vi "Lab5_template_v4.0.vi"() -> ()   [LabVIEW 2018]
doc: "Main VI for the controls"
uses:
  components/PMCL Dynamic Signal Analyzer/Controls/DSA excitation specs.ctl
  components/PMCL Dynamic Signal Analyzer/Controls/DSA cycle specs.ctl
  Typedefs/StateDef_Enum.ctl
  <vilib>/Utility/error.llb/DialogType.ctl
  <vilib>/Platform/TimedLoop/XDataNode/timing_clust.ctl
  <vilib>/Platform/TimedLoop/XDataNode/nitl_modes.ctl
  <vilib>/Platform/TimedLoop/XDataNode/wakeup.ctl
  <vilib>/DAQmx/read.llb/DAQmx Read (Analog 1D DBL NChan 1Samp).vi
  <vilib>/DAQmx/write.llb/DAQmx Write (Analog DBL 1Chan 1Samp).vi
  <vilib>/DAQmx/create/channels.llb/DAQmx Create Channel (AO-Voltage-Basic).vi
  <vilib>/DAQmx/create/channels.llb/DAQmx Create Channel (AI-Voltage-Basic).vi
  <vilib>/DAQmx/configure/timing.llb/DAQmx Timing (Sample Clock).vi
  <vilib>/DAQmx/create/timing.llb/DAQmx Create Timing Source (Control Loop From Task).vi
  <vilib>/DAQmx/miscellaneous.llb/DAQmx Fill In Error Info.vi
  <vilib>/platform/TimedLoop/XDataNode/XDataNode.xnode
  Components/Timing/Timing.lvlib
  <vilib>/Platform/TimedLoop/XDataNode/XDNodeRunTimeDep.lvlib
  <vilib>/Analysis/NI_AALPro.lvlib
  <vilib>/ptbypt/NI_PtbyPt.lvlib
  Components/Controller/Controller.lvlib
panel:
  in  "System Stop Button":bool
  in  "Pause chart?":bool
  in  "Controller Params":enum32{"Page 1"}(tab)
  in  "Kp":dbl=1.0 min=0.0
  in  "Controller On?":bool
  out "Status":string
  in  "Ref. Gen.":enum32{"Analog In", "Manual", "Wave Gen", "DSA"}(tab)=enum."Manual"
  in  "Ref. cmd.":dbl(slide) step=1.0 scale=-10.0..10.0 scale format="%#.1f"
  in  "Signal Cluster":T1={"phase"=0.0, "amplitude"=1.0, "frequency"=1.0, "offset"=1.0, "Signal"=enum."Square"} {"offset" format="%0.2f"; "frequency" format="%0.2f"; "amplitude" format="%0.2f"; "phase" format="%0.2f"}
  in  "Frequency\nResponse":enum16{"Plant", "RR", "CL"}(ring)
  out "DSA \nRunning?":bool
  in  "Stop \nDSA":bool
  in  "Start \nDSA":bool
  in  "DSA excitation specs":T2={"Initial Freq. [Hz]"=10.0, "Final Freq. [Hz]"=999.0, "# pts. in interval"=50, "Samping Time [s]"=0.001, "Amplitude [V]"=1.0, "Offset [V]"=0.0, "Freq Units (F: rad/s, T: Hz)"=TRUE}
  in  "Cycle Specs":T3={"Cycles To \nSettle (M)"=5, "Cycles To \nCalculate (N)"=10}
  in  "Loop Timing":enum32{"Ctrl.", "Ref. gen", "UI"}(tab)
  in  "Ctrl.\nLoop Rate (Hz)":dbl=20000.0 format="%#_4p"
  out "# Finished\nLate counter":dbl
  out "# Finished\nLate counter":dbl
  in  "Ref. Gen.\nLoop Rate (Hz)":dbl=20000.0 format="%#_4p"
  in  "UI Loop rate (Hz)":dbl=1000.0 format="%#_6p"
  in  "Display Waveforms":enum32{"Controller Signals", "DSA "}(tab)
  out "Control Effort":dbl(graph)
  out "Waveform Chart":cluster{"Double":dbl, "Numeric":dbl}(graph)
  out "Phase Bode Plot":cluster{dbl[], dbl[]}(graph)
  out "Magnitude Bode Plot":cluster{dbl[], dbl[]}(graph)
  out "DSA Signals":cluster{"Double":dbl, "Double":dbl}(graph)
  # "Connect the Reference Signal \nto C/AI 1 of the myRIO."
  # "Pinout Config.:\nPort C/AI0 : Plant output being read           by the controller.\nPort C/AI1 : Reference signal for the control loop.\nPort C/AO0 : Control effort signal to the plant."
  # "Control Loop Timing"
  # "Ref.  Gen. Loop Timing"
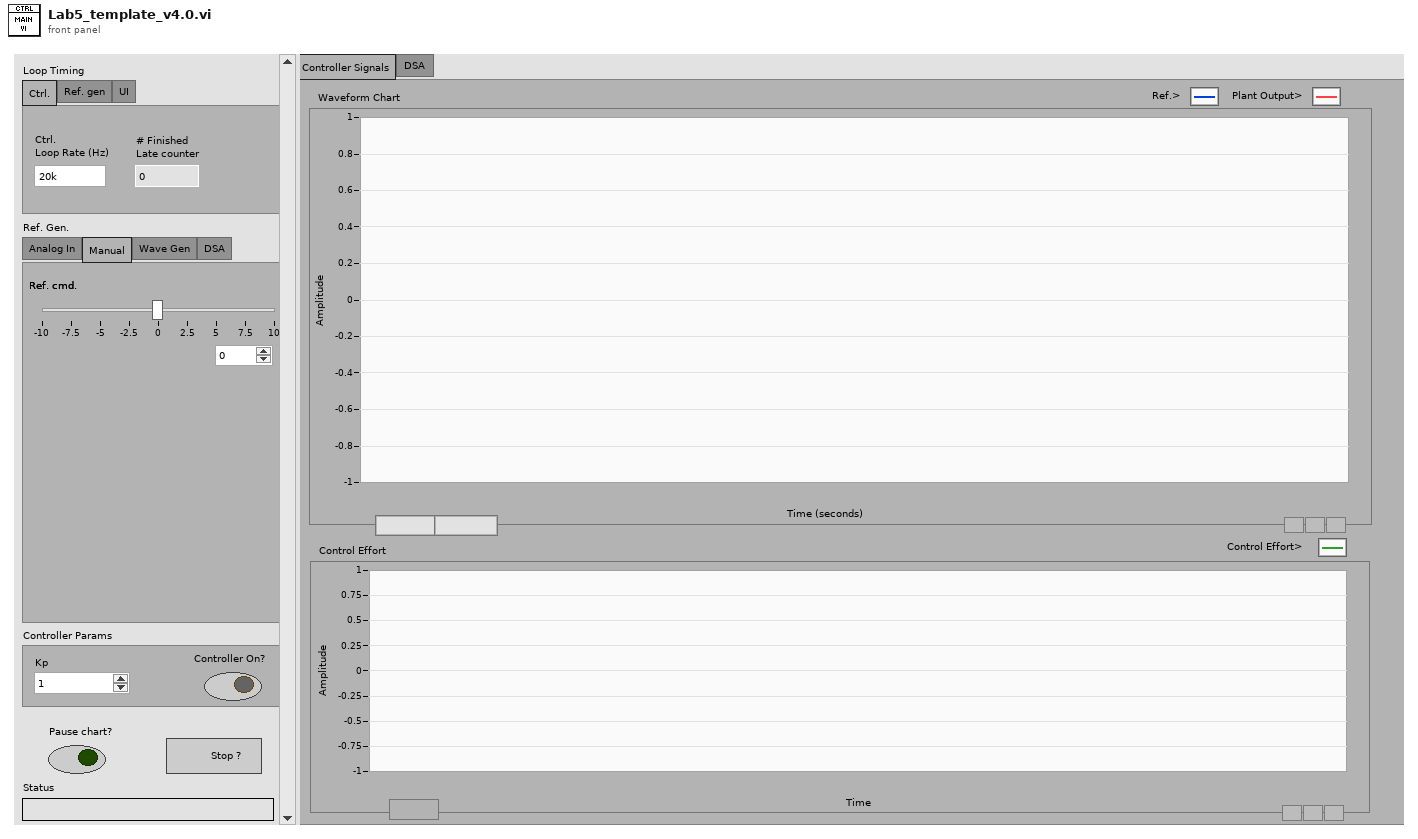
[diagram p1: front panel]
types:
  T1 = cluster{"phase":dbl, "amplitude":dbl, "frequency":dbl, "offset":dbl, "Signal":enum16{"Sine", "Square", "Sawtooth"}}
  T2 = typedef "DSA excitation specs.ctl" = cluster{"Initial Freq. [Hz]":dbl, "Final Freq. [Hz]":dbl, "# pts. in interval":i16, "Samping Time [s]":dbl, "Amplitude [V]":dbl, "Offset [V]":dbl, "Freq Units (F: rad/s, T: Hz)":bool}
  T3 = typedef "DSA cycle specs.ctl" = cluster{"Cycles To \nSettle (M)":i16, "Cycles To \nCalculate (N)":i16}
  T4 = typedef "DialogType.ctl" = u16
  T5 = typedef "StateDef_Enum.ctl" = enum16{"Initialize", "Wait", "Shutdown"}
  T6 = typedef "XDNodeRunTimeDep.lvlib/timing_clust.ctl" = cluster{"Expected End [f-1]":u64, "Actual End [f-1]":u64, "Finished Late? [f-1]":bool, "Expected End [i-1]":u64, "Actual End [i-1]":u64, "Finished Late? [i-1]":bool, "Expected Start [i]":u64, "Actual Start [i]":u64, "Expected Start [f]":u64, "Actual Start [f]":u64, "Source Name":string, "Structure Name":string, "Period":i64, "Deadline":i64, "Offset":i64, "Start":i64, "Priority":i32, "Timeout":i32, "Mode":T7, "Wakeup Reason":T8, "Error":errorcluster, "Source Type":string, "Secondary Source Type":string, "Global End Time":u64, "Global Start Time":u64, "Frame Duration":u64, "Iteration Duration":u64, "Assigned CPU":i32, "I/O Scan Engine Mode":u32}
  T7 = typedef "XDNodeRunTimeDep.lvlib/nitl_modes.ctl" = enum32{"No Change", "Process missed periods, maintain original phase", "Discard missed periods, maintain original phase", "Process missed periods, ignore original phase", "Discard missed periods, ignore original phase"}
  T8 = typedef "XDNodeRunTimeDep.lvlib/wakeup.ctl" = enum32{"Normal", "Aborted", "Asynchronous wakeup", "Timing source error", "Timed loop error", "Timeout"}
  T9 = cluster{"Analog In CH1":dbl, "Analog In CH0":dbl}
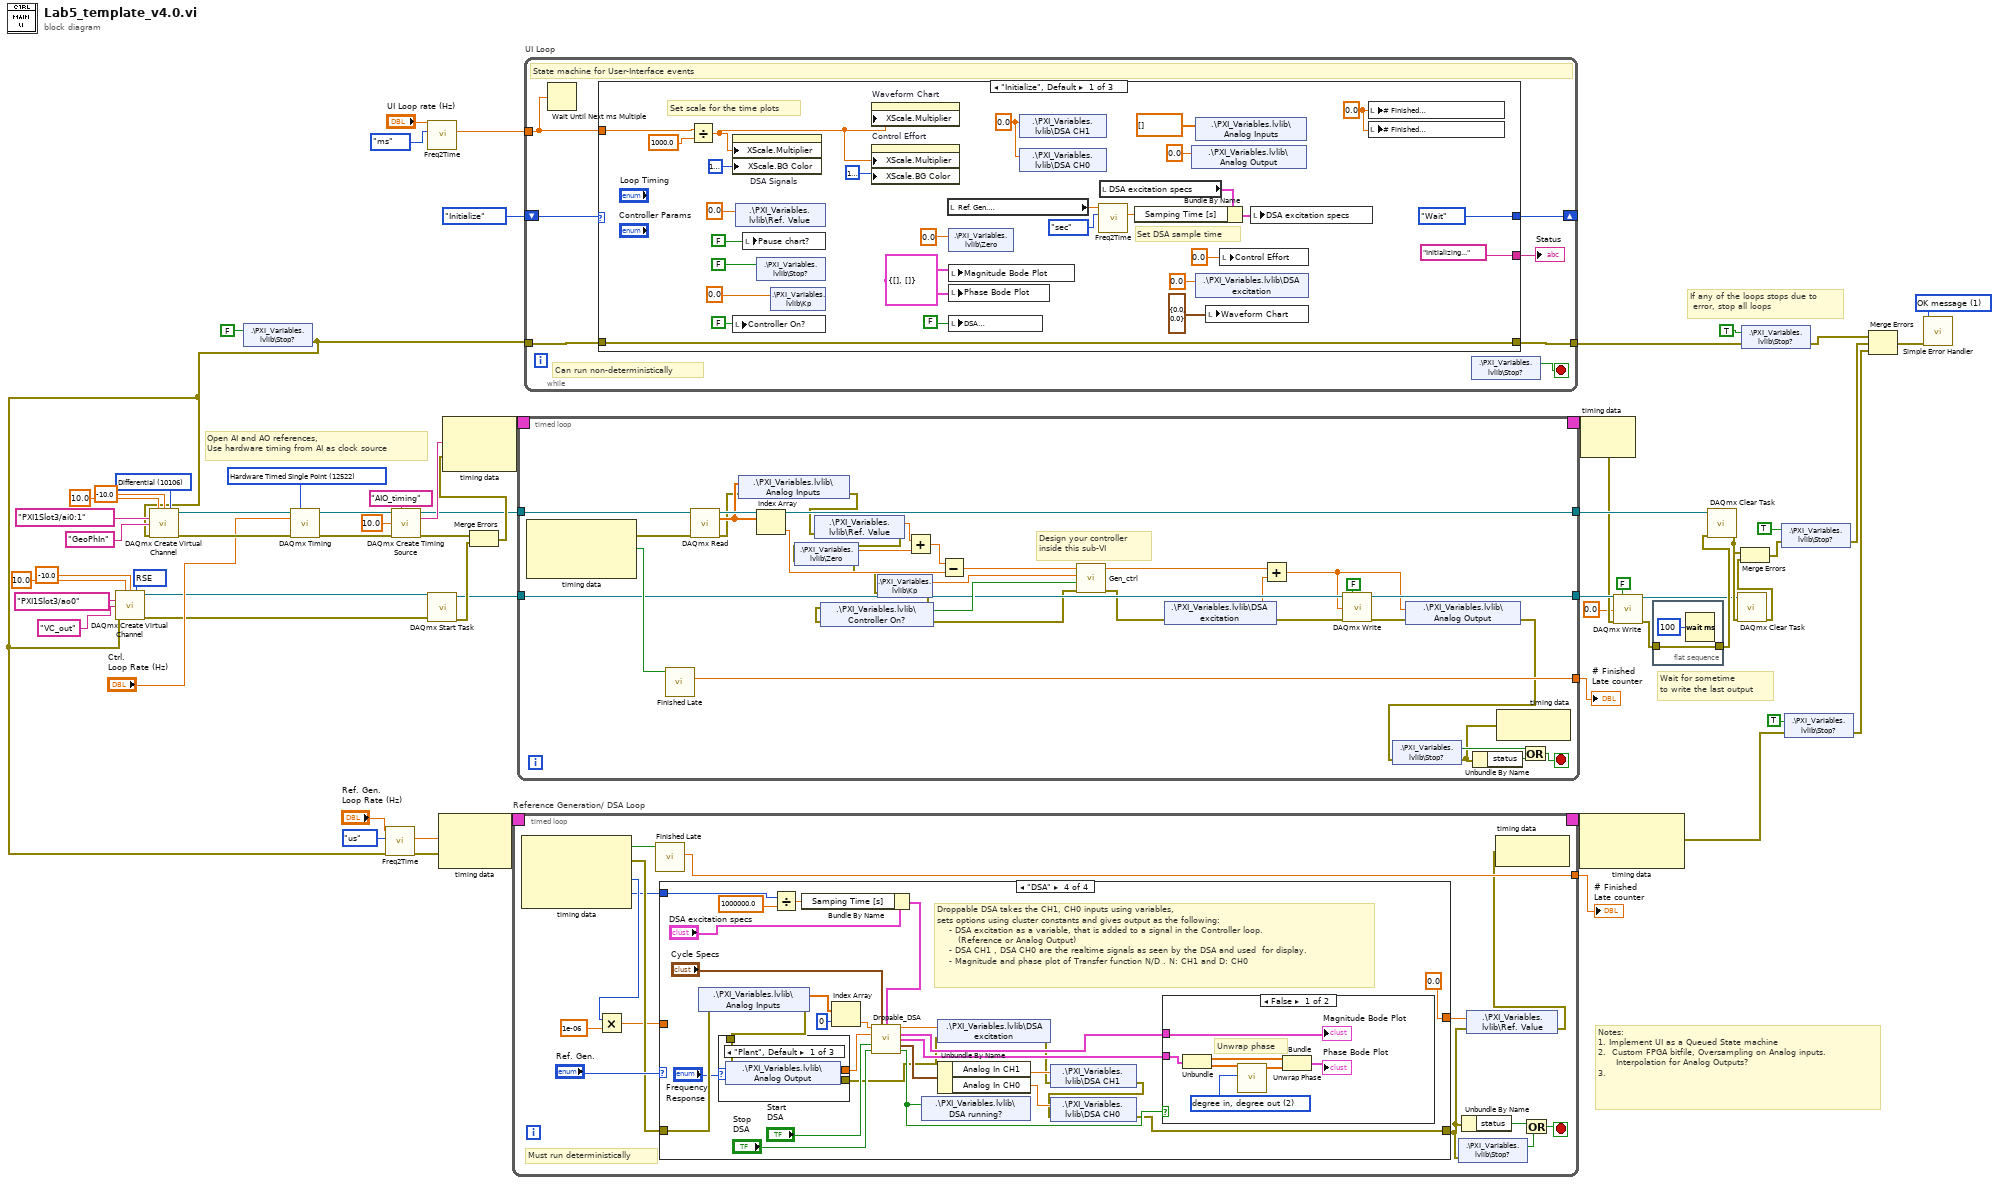
[diagram p0: block diagram]
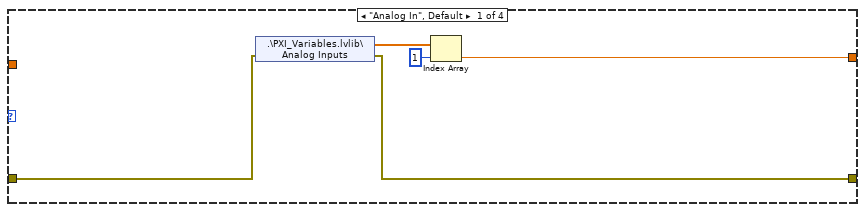
[diagram p2: hidden frame]
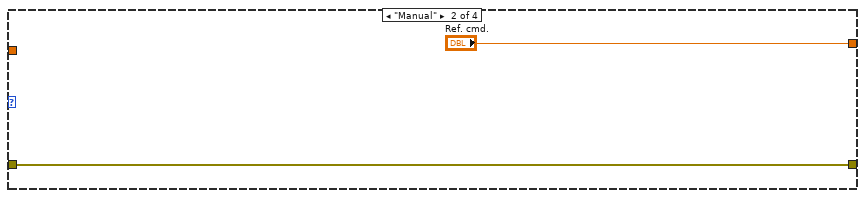
[diagram p3: hidden frame]
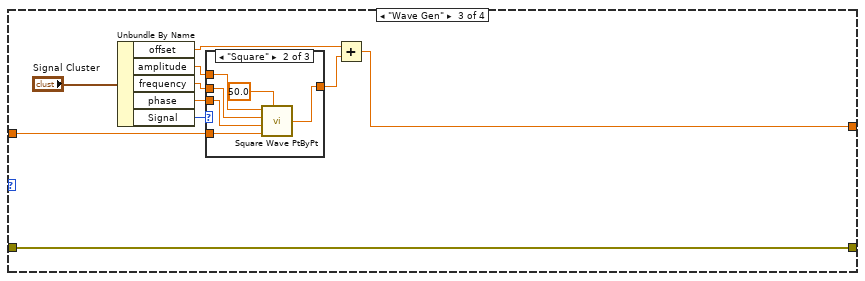
[diagram p4: hidden frame]
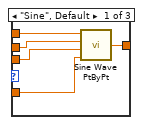
[diagram p5: hidden frame]
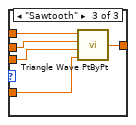
[diagram p6: hidden frame]
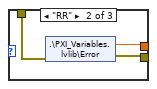
[diagram p7: hidden frame]
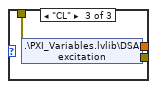
[diagram p8: hidden frame]
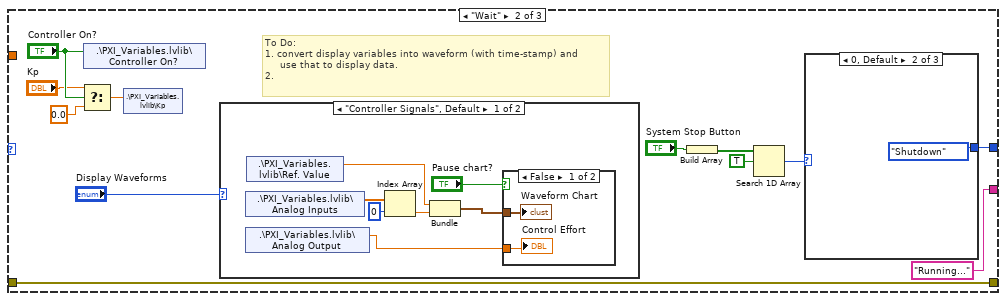
[diagram p10: hidden frame]
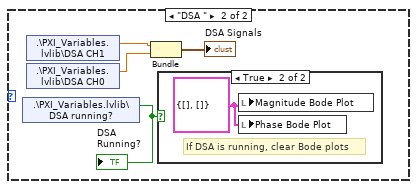
[diagram p12: hidden frame]
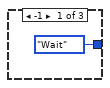
[diagram p14: hidden frame]
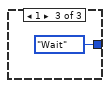
[diagram p15: hidden frame]
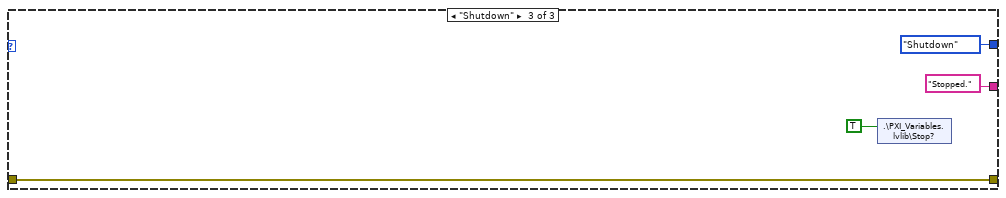
[diagram p16: hidden frame]
diagram:
  w19 = T4 1 items=["no dialog", "OK message", "continue or stop message", "OK message + warnings", "continue/stop + warnings"] ("type of dialog (OK msg:1)")
  w25 = 12522 items=["Finite Samples"=10178, "Continuous Samples"=10123, "Hardware Timed Single Point"=12522] ("sample mode")
  w42 = 10106 items=["Default"=-1, "RSE"=10083, "NRSE"=10078, "Differential"=10106, "Pseudodifferential"=12529] ("input terminal configuration")
  w46 = 10083 items=["Default"=-1, "RSE"=10083, "Differential"=10106, "Pseudodifferential"=12529] ("output terminal configuration")
  # "Wait for sometime \nto write the last output"
  # "Open AI and AO references,\nUse hardware timing from AI as clock source"
  # "Notes:\n1. Implement UI as a Queued State machine\n2.  Custom FPGA bitfile, Oversampling on Analog inputs. \n      Interpolation for Analog Outputs?\n3."
  # "If any of the loops stops due to\n error, stop all loops"
  n1 = shared-variable ".\\PXI_Variables.lvlib\\Stop?"(FALSE ("Stop?")) -> (error out=w1:errorcluster)  [unwired: 1 in]
  n2 = call-poly <vilib>:"DAQmx Create Virtual Channel.vi"("maximum value"=10.0, "minimum value"=-10.0, "output terminal configuration"=w46, "physical channels"=tag "PXI1Slot3/ao0", "name to assign"="VC_out", "error in"=w1) -> ("task out"=w4:refnum<k21>, "error out"=w3:errorcluster)  [unwired: 8 in]
  n3 = call-poly <vilib>:"DAQmx Create Virtual Channel.vi"("maximum value"=10.0, "minimum value"=-10.0, "input terminal configuration"=w42, "physical channels"=tag "PXI1Slot3/ai0:1", "name to assign"="GeoPhIn", "error in"=w1) -> ("task out"=w27:refnum<k21>, "error out"=w26:errorcluster)  [unwired: 8 in]
  n4 = call-poly <vilib>:"DAQmx Timing.vi"("task/channels in"=w27, "sample mode"=w25, "rate"="Ctrl.\nLoop Rate (Hz)", "error in"=w26) -> ("task out"=w20:refnum<k21>, "error out"=w22:errorcluster)  [unwired: 10 in]
  n5 = call "Freq2Time.vi"("error in (no error)"=w1, "Int. Time Unit"=enum16{"sec", "us", "ms"}."us", "Sample rate (Hz)"="Ref. Gen.\nLoop Rate (Hz)") -> ("error out"=w2:errorcluster, "Int.  time [unit]"=w17:dbl)  [unwired: 6 in, 1 out]
  n6 = call-poly <vilib>:"DAQmx Create Timing Source.vi"("task/channels in"=w20, "timing source name"="AIO_timing", "sleep time (us)"=10.0, "error in"=w22) -> ("task out"=w23:refnum<k21>, "timing source out"=w24:string, "error out"=w21:errorcluster)  [unwired: 9 in]
  n7 = call "Freq2Time.vi"("Int. Time Unit"=enum16{"sec", "us", "ms"}."ms", "Sample rate (Hz)"="UI Loop rate (Hz)") -> ("Int.  time [unit]"=w54:dbl)  [unwired: 7 in, 2 out]
  n8 = call <vilib>:"DAQmx Start Task.vi"("task/channels in"=w4, "error in"=w3) -> ("task out"=w28:refnum<k21>, "error out"=w44:errorcluster)  [unwired: 12 in]
  n9 = node-c288(w17, w2) -> (w61:T6)
  n10 = Merge Errors(w21, w44) -> (w36:errorcluster)
  n11 = node-c288(w24, w36) -> (w38:T6)
  n12 = timed-loop "Reference Generation/ DSA Loop" {
    timing: w61 -> [_]
    timing-out: [_] -> w60
    tunnel: [w76] -> w59
    stop <- w70 stop-if-true
    # "Must run deterministically"
    n13 = node-c288() -> (w77:bool, w73:errorcluster, w67:i64, w66:i64)  [unwired: 1 in]
    n14 = Multiply(x=w67, y=1e-06) -> (x*y=w69:dbl)
    n15 = call "Finished Late.vi"("Finished \nLate?"=w77) -> ("# Finished\nLate counter"=w76:dbl)  [unwired: 8 in, 2 out]
    n16 = case shown="\"DSA\"" "Ref. Gen." {
      tunnel: [w82 "Ref. cmd." w87 0.0 ("Ref. cmd.")] -> w74
      tunnel: w73 -> [w80 w83 w86 w117]
      tunnel: [w79 w83 w86 w120] -> w64
      tunnel: w69 -> [_ _ w85 _]
      tunnel: w66 -> [_ _ _ w127]
      frame "Analog In", Default {
        n17 = shared-variable ".\\PXI_Variables.lvlib\\Analog Inputs"(error in=w80) -> (w81:dbl[], error out=w79:errorcluster)
        n18 = Index Array(array=w81, index=1) -> (element=w82:dbl)
      }
      frame "Manual" {
      }
      frame "Wave Gen" {
        n19 = Unbundle By Name("Signal Cluster") -> ("offset"=w88:dbl, "amplitude"=w91:dbl, "frequency"=w90:dbl, "phase"=w89:dbl, "Signal"=w92:enum16{"Sine", "Square", "Sawtooth"})
        n20 = case shown="\"Square\"" w92 {
          tunnel: [w99 w104 w110] -> w94
          tunnel: w91 -> [w98 w103 w109]
          tunnel: w90 -> [w97 w102 w108]
          tunnel: w89 -> [w96 w101 w107]
          tunnel: w85 -> [w95 w100 w106]
          frame "Sine", Default {
            n21 = call <vilib>:"Sine Wave PtByPt.vi"("time"=w95, "phase"=w96, "frequency"=w97, "amplitude"=w98) -> ("sine wave"=w99:dbl)
          }
          frame "Square" {
            n22 = call <vilib>:"Square Wave PtByPt.vi"("amplitude"=w103, "frequency"=w102, "phase"=w101, "time"=w100, "duty cycle (%)"=50.0) -> ("square wave"=w104:dbl)
          }
          frame "Sawtooth" {
            n23 = call <vilib>:"Triangle Wave PtByPt.vi"("time"=w106, "phase"=w107, "frequency"=w108, "amplitude"=w109) -> ("triangle wave"=w110:dbl)
          }
        }
        n24 = Add(x=w88, y=w94) -> (x+y=w87:dbl)
      }
      frame "DSA" {
        # "Droppable DSA takes the CH1, CH0 inputs using variables, \nsets options using cluster constants and gives output as the following:\n    - DSA excitation as a variable, that is added to a signal in the Controller loop. \n       (Reference or Analog Output)\n    - DSA CH1 , DSA CH0 are the realtime signals as seen by the DSA and used  for display.\n    - Magnitude and phase plot of Transfer function N/D . N: CH1 and D: CH0"
        n25 = shared-variable ".\\PXI_Variables.lvlib\\Analog Inputs"(error in=w117) -> (w116:dbl[], error out=w114:errorcluster)
        n26 = case shown="\"Plant\", Default" "Frequency\nResponse" {
          tunnel: [w140 w143 w144] -> w115
          tunnel: w114 -> [w139 w141 w146]
          tunnel: [w138 w142 w145] -> w111
          frame "Plant", Default {
            n27 = shared-variable ".\\PXI_Variables.lvlib\\Analog Output"(error in=w139) -> (w140:dbl, error out=w138:errorcluster)
          }
          frame "RR" {
            n28 = shared-variable ".\\PXI_Variables.lvlib\\Error"(error in=w141) -> (w143:dbl, error out=w142:errorcluster)
          }
          frame "CL" {
            n29 = shared-variable ".\\PXI_Variables.lvlib\\DSA excitation"(error in=w146) -> (w144:dbl, error out=w145:errorcluster)
          }
        }
        n30 = Divide(x=w127, y=1000000.0) -> (x/y=w125:dbl)
        n31 = Bundle By Name(cluster="DSA excitation specs", "Samping Time [s]"=w125) -> (w124:T2)
        n32 = Index Array(array=w116, index=0) -> (element=w118:dbl)
        n33 = call "Dropable_DSA.vi"("Analog In CH1"=w118, "Cycle Specs"="Cycle Specs", "Excitation Specs"=w124, "Analog In CH0"=w115, "START"="Start \nDSA", "STOP"="Stop \nDSA") -> ("Analog Out"=w136:dbl, "Bode Magnitude"=w129:cluster{dbl[], dbl[]}, "Bode Phase"=w128:cluster{dbl[], dbl[]}, "Live signals"=w133:T9, "Running"=w123:bool)  [unwired: 4 in, 1 out]
        n34 = shared-variable ".\\PXI_Variables.lvlib\\DSA running?"(w123) -> ()  [unwired: 1 in, 1 out]
        n35 = shared-variable ".\\PXI_Variables.lvlib\\DSA excitation"(w136, error in=w111) -> (error out=w122:errorcluster)
        n36 = Unbundle By Name(w133) -> ("Analog In CH1"=w132:dbl, "Analog In CH0"=w131:dbl)
        n37 = shared-variable ".\\PXI_Variables.lvlib\\DSA CH1"(w132, error in=w122) -> (error out=w121:errorcluster)
        n38 = shared-variable ".\\PXI_Variables.lvlib\\DSA CH0"(w131, error in=w121) -> (error out=w120:errorcluster)
        n39 = case shown="False" w123 {
          tunnel: w129 -> [w147 _]
          tunnel: w128 -> [w149 _]
          frame False {
            w151 = 2 items=["radian in, radian out", "radian in, degree out", "degree in, degree out", "degree in, radian out"] ("phase unit")
            # "Unwrap phase"
            n40 = Unbundle(w149) -> (w153:dbl[], w150:dbl[])
            n41 = call <vilib>:"Unwrap Phase.vi"("phase unit"=w151, "Phase"=w150) -> ("Unwrapped Phase"=w152:dbl[])  [unwired: 8 in, 1 out]
            n42 = Bundle(w153, "Unwrapped Phase"=w152) -> (→"Phase Bode Plot":cluster{dbl[], "Unwrapped Phase":dbl[]})  [unwired: 1 in]
            "Magnitude Bode Plot" <- w147
          }
          frame True {
          }
        }
      }
    }
    n43 = shared-variable ".\\PXI_Variables.lvlib\\Stop?"(error in=w64) -> (w71:bool)  [unwired: 1 out]
    n44 = Unbundle By Name(w64) -> ("status"=w72:bool)
    n45 = shared-variable ".\\PXI_Variables.lvlib\\Ref. Value"(w74, error in=w64) -> (error out=w65:errorcluster)
    n46 = node-c288(w65) -> ()  [unwired: 1 out]
    n47 = Or(x=w72, y=w71) -> (x .or. y?=w70:bool)
  }
  "# Finished\nLate counter" <- w59
  n48 = timed-loop {
    timing: w38 -> [_]
    timing-out: [_] -> w37
    tunnel: w23 -> [w193]
    tunnel: [w191] -> w30
    tunnel: [w190] -> w29
    tunnel: w28 -> [w177]
    tunnel: [w176] -> w11
    stop <- w178 stop-if-true
    # "Design your controller \ninside this sub-VI"
    n49 = node-c288() -> (w194:errorcluster, w192:bool)  [unwired: 1 in, 1 out]
    n50 = call "Finished Late.vi"("Finished \nLate?"=w192) -> ("# Finished\nLate counter"=w191:dbl)  [unwired: 8 in, 2 out]
    n51 = call-poly <vilib>:"DAQmx Read.vi"("task/channels in"=w193, "error in"=w194) -> ("task out"=w190:refnum<k21>, "data"=w189:dbl[], "error out"=w174:errorcluster)  [unwired: 11 in]
    n52 = shared-variable ".\\PXI_Variables.lvlib\\Analog Inputs"(w189, error in=w174) -> (error out=w173:errorcluster)
    n53 = Index Array(array=w189) -> (element=w188:dbl)  [unwired: 1 in]
    n54 = shared-variable ".\\PXI_Variables.lvlib\\Ref. Value"(error in=w173) -> (w186:dbl, error out=w172:errorcluster)
    n55 = shared-variable ".\\PXI_Variables.lvlib\\Zero"(error in=w172) -> (w185:dbl, error out=w171:errorcluster)
    n56 = shared-variable ".\\PXI_Variables.lvlib\\Kp"(error in=w171) -> (w183:dbl, error out=w170:errorcluster)
    n57 = shared-variable ".\\PXI_Variables.lvlib\\Controller On?"(error in=w170) -> (w182:bool, error out=w169:errorcluster)
    n58 = Add(x=w186, y=w185) -> (x+y=w187:dbl)
    n59 = Subtract(x=w187, y=w188) -> (x-y=w184:dbl)
    n60 = call "Gen_ctrl.vi"("error in (no error)"=w169, "Controller On?"=w182, "Kp"=w183, "Error In"=w184) -> ("error out"=w168:errorcluster, "Ctrl Effort Out"=w166:dbl)  [unwired: 6 in]
    n61 = shared-variable ".\\PXI_Variables.lvlib\\DSA excitation"(error in=w168) -> (w165:dbl, error out=w167:errorcluster)
    n62 = Add(x=w166, y=w165) -> (x+y=w175:dbl)
    n63 = call-poly <vilib>:"DAQmx Write.vi"("task/channels in"=w177, "auto start"=FALSE, "data"=w175, "error in"=w167) -> ("task out"=w176:refnum<k21>, "error out"=w164:errorcluster)  [unwired: 9 in, 1 out]
    n64 = shared-variable ".\\PXI_Variables.lvlib\\Analog Output"(w175, error in=w164) -> (error out=w163:errorcluster)
    n65 = shared-variable ".\\PXI_Variables.lvlib\\Stop?"(error in=w163) -> (w181:bool, error out=w180:errorcluster)
    n66 = Unbundle By Name(w180) -> ("status"=w179:bool)
    n67 = node-c288(w180) -> ()  [unwired: 1 out]
    n68 = Or(x=w181, y=w179) -> (x .or. y?=w178:bool)
  }
  "# Finished\nLate counter" <- w30
  n69 = while "UI Loop" {
    shift-right: [w206] -> _
    shift-left: StateDef_Enum."Initialize" ("State defining Enum") -> [w207]
    tunnel: w1 -> [w205]
    tunnel: [w204] -> w53
    tunnel: w54 -> [w201]
    stop <- w202 stop-if-true
    # "Can run non-deterministically"
    # "State machine for User-Interface events"
    n70 = Wait Until Next ms Multiple(millisecond multiple=w201) -> ()  [unwired: 1 out]
    n71 = case shown="\"Initialize\", Default" w207 {
      tunnel: [StateDef_Enum."Wait" ("State defining Enum") w244 StateDef_Enum."Shutdown" ("State defining Enum")] -> w206
      tunnel: w205 -> [w232 w242 w268]
      tunnel: [w232 w242 w268] -> w204
      tunnel: ["Initializing..." ("Status") "Running..." ("Status") "Stopped." ("Status")] -> w203
      tunnel: w201 -> [w230 _ _]
      frame "Initialize", Default {
        w208 = 0.0 ("# Finished\nLate counter")
        w209 = 0.0 ("DSA CH1")
        w225 = cluster{dbl[], dbl[]} {[], []} ("Magnitude Bode Plot")
        # "Set DSA sample time"
        # "Set scale for the time plots"
        n72 = Divide(x=w230, y=1000.0) -> (x/y=w217:dbl)
        n73 = property on="DSA Signals" class="WFChart (strict)"("XScale.Multiplier"=w217, "XScale.BG Color"=u32 16777216) -> ()  [unwired: 2 in, 2 out]
        n74 = local write "Controller On?"(FALSE ("Controller On?")) -> ()
        n75 = shared-variable ".\\PXI_Variables.lvlib\\Ref. Value"(0.0 ("Ref. Value")) -> ()  [unwired: 1 in, 1 out]
        n76 = local write "Pause chart?"(FALSE ("Pause chart?")) -> ()
        n77 = shared-variable ".\\PXI_Variables.lvlib\\Stop?"(FALSE ("Stop?")) -> ()  [unwired: 1 in, 1 out]
        n78 = shared-variable ".\\PXI_Variables.lvlib\\Kp"(0.0 ("Kp")) -> ()  [unwired: 1 in, 1 out]
        n79 = property on="Waveform Chart" class="WFChart (strict)"("XScale.Multiplier"=w217) -> ()  [unwired: 2 in, 2 out]
        n80 = property on="Control Effort" class="WFChart (strict)"("XScale.Multiplier"=w217, "XScale.BG Color"=u32 16777216) -> ()  [unwired: 2 in, 2 out]
        n81 = local read "Ref. Gen.\nLoop Rate (Hz)"() -> (w220:dbl)
        n82 = shared-variable ".\\PXI_Variables.lvlib\\Zero"(0.0 ("Zero")) -> ()  [unwired: 1 in, 1 out]
        n83 = local write "Magnitude Bode Plot"(w225) -> ()
        n84 = local write "Phase Bode Plot"(w225) -> ()
        n85 = local write "DSA \nRunning?"(FALSE ("DSA \nRunning?")) -> ()
        n86 = shared-variable ".\\PXI_Variables.lvlib\\DSA CH1"(w209) -> ()  [unwired: 1 in, 1 out]
        n87 = shared-variable ".\\PXI_Variables.lvlib\\DSA CH0"(w209) -> ()  [unwired: 1 in, 1 out]
        n88 = call "Freq2Time.vi"("Int. Time Unit"=enum16{"sec", "us", "ms"}."sec", "Sample rate (Hz)"=w220) -> ("Int.  time [unit]"=w218:dbl)  [unwired: 7 in, 2 out]
        n89 = local read "DSA excitation specs"() -> (w222:T2)
        n90 = Bundle By Name(cluster=w222, "Samping Time [s]"=w218) -> (w221:T2)
        n91 = shared-variable ".\\PXI_Variables.lvlib\\Analog Output"(0.0 ("Analog Output")) -> ()  [unwired: 1 in, 1 out]
        n92 = shared-variable ".\\PXI_Variables.lvlib\\Analog Inputs"(dbl[] [] ("Analog Inputs")) -> ()  [unwired: 1 in, 1 out]
        n93 = shared-variable ".\\PXI_Variables.lvlib\\DSA excitation"(0.0 ("DSA excitation")) -> ()  [unwired: 1 in, 1 out]
        n94 = local write "Waveform Chart"(cluster{"Double":dbl, "Numeric":dbl} {"Double"=0.0, "Numeric"=0.0} ("Waveform Chart")) -> ()
        n95 = local write "Control Effort"(0.0 ("Control Effort")) -> ()
        n96 = local write "DSA excitation specs"(w221) -> ()
        n97 = local write "# Finished\nLate counter"(w208) -> ()
        n98 = local write "# Finished\nLate counter"(w208) -> ()
      }
      frame "Wait" {
        # "To Do:\n1. convert display variables into waveform (with time-stamp) and\n     use that to display data.\n2."
        n99 = Select(t="Kp", s="Controller On?", f=0.0) -> (s? t:f=w240:dbl)
        n100 = shared-variable ".\\PXI_Variables.lvlib\\Controller On?"("Controller On?") -> ()  [unwired: 1 in, 1 out]
        n101 = shared-variable ".\\PXI_Variables.lvlib\\Kp"(w240) -> ()  [unwired: 1 in, 1 out]
        n102 = case shown="\"Controller Signals\", Default" "Display Waveforms" {
          frame "Controller Signals", Default {
            n103 = shared-variable ".\\PXI_Variables.lvlib\\Analog Inputs"() -> (w254:dbl[])  [unwired: 1 in, 1 out]
            n104 = shared-variable ".\\PXI_Variables.lvlib\\Analog Output"() -> (w248:dbl)  [unwired: 1 in, 1 out]
            n105 = shared-variable ".\\PXI_Variables.lvlib\\Ref. Value"() -> (w251:dbl)  [unwired: 1 in, 1 out]
            n106 = Index Array(array=w254, index=0) -> (element=w253:dbl)
            n107 = Bundle("Double"=w251, "Numeric"=w253) -> (w249:cluster{"Double":dbl, "Numeric":dbl})  [unwired: 1 in]
            n108 = case shown="False" "Pause chart?" {
              tunnel: w249 -> [w256 _]
              tunnel: w248 -> [w255 _]
              frame False {
                "Waveform Chart" <- w256
                "Control Effort" <- w255
              }
              frame True {
              }
            }
          }
          frame "DSA " {
            n109 = shared-variable ".\\PXI_Variables.lvlib\\DSA running?"() -> (w257:bool)  [unwired: 1 in, 1 out]
            "DSA \nRunning?" <- w257
            n110 = shared-variable ".\\PXI_Variables.lvlib\\DSA CH1"() -> (w259:dbl)  [unwired: 1 in, 1 out]
            n111 = shared-variable ".\\PXI_Variables.lvlib\\DSA CH0"() -> (w258:dbl)  [unwired: 1 in, 1 out]
            n112 = Bundle("Double"=w259, "Double"=w258) -> (→"DSA Signals":cluster{"Double":dbl, "Double":dbl})  [unwired: 1 in]
            n113 = case shown="True" w257 {
              frame False {
              }
              frame True {
                w261 = cluster{dbl[], dbl[]} {[], []} ("Magnitude Bode Plot")
                # "If DSA is running, clear Bode plots"
                n114 = local write "Magnitude Bode Plot"(w261) -> ()
                n115 = local write "Phase Bode Plot"(w261) -> ()
              }
            }
          }
        }
        n116 = Build Array("System Stop Button") -> (w246:bool[])
        n117 = Search 1D Array(1D array=w246, element=TRUE) -> (index of element=w243:i32)  [unwired: 1 in]
        n118 = case shown="0, Default" w243 {
          tunnel: [StateDef_Enum."Wait" ("State defining Enum") StateDef_Enum."Shutdown" ("State defining Enum") StateDef_Enum."Wait" ("State defining Enum")] -> w244
          frame -1 {
          }
          frame 0, Default {
          }
          frame 1 {
          }
        }
      }
      frame "Shutdown" {
        n119 = shared-variable ".\\PXI_Variables.lvlib\\Stop?"(TRUE) -> ()  [unwired: 1 in, 1 out]
      }
    }
    "Status" <- w203
    n120 = shared-variable ".\\PXI_Variables.lvlib\\Stop?"() -> (w202:bool)  [unwired: 1 in, 1 out]
  }
  n121 = node-c288(w60) -> (w58:errorcluster)  [unwired: 1 out]
  n122 = node-c288(w37) -> (w10:errorcluster)
  n123 = call-poly <vilib>:"DAQmx Write.vi"("task/channels in"=w11, "auto start"=FALSE, "data"=0.0, "error in"=w10) -> ("task out"=w6:refnum<k21>, "error out"=w8:errorcluster)  [unwired: 9 in, 1 out]
  n124 = flat-sequence {
    tunnel: [w270] -> w7
    tunnel: w8 -> [w270]
    frame #0 {
      n125 = Wait (ms)(milliseconds to wait=u32 100) -> ()  [unwired: 1 out]
    }
  }
  n126 = call <vilib>:"DAQmx Clear Task.vi"("task in"=w29, "error in"=w7) -> ("error out"=w13:errorcluster)  [unwired: 13 in]
  n127 = call <vilib>:"DAQmx Clear Task.vi"("task in"=w6, "error in"=w13) -> ("error out"=w33:errorcluster)  [unwired: 13 in]
  n128 = Merge Errors(w13, w33) -> (w34:errorcluster)
  n129 = shared-variable ".\\PXI_Variables.lvlib\\Stop?"(TRUE ("Stop?"), error in=w53) -> (error out=w52:errorcluster)
  n130 = shared-variable ".\\PXI_Variables.lvlib\\Stop?"(TRUE ("Stop?"), error in=w34) -> (error out=w31:errorcluster)
  n131 = shared-variable ".\\PXI_Variables.lvlib\\Stop?"(TRUE ("Stop?"), error in=w58) -> (error out=w32:errorcluster)
  n132 = Merge Errors(w52, w31, w32) -> (w62:errorcluster)
  n133 = call <vilib>:"Simple Error Handler.vi"("type of dialog (OK msg:1)"=w19, "error in (no error)"=w62) -> ()  [unwired: 3 in, 5 out]
